vi "DualDigitalOscilloscope .vi"() -> ()   [LabVIEW 2014]
panel:
  out "error out":errorcluster
  in  "Digitalizing Parameters":T1={"Number of Samples"=500.0, "Sampling Frequency"=10000.0}
  out "Waveform Graph":dynamicdata(graph)=[{"t0"=timestamp(3496344962.5394974 s since 1904-01-01), "dt"=0.001, "Y"=[-8.590041558292159, -8.440717982918141, -8.128256863855041, -7.667459197369262, -7.046484650384645, -6.271253896732339, -5.352621206174619, -4.313939189246366, -3.190071979714034, -2.0010828273437613, -0.7699949874285559, 0.4729325219573479, 1.7063211765178325, 2.9114237139782557, 4.057652341722364, 5.131522209673436, 6.100800901298043, 6.935887140374739, 7.623953652074697, 8.147897360293387, 8.511665011024219, 8.741897737995128, 8.794851269409115, 8.618229869568173, 8.298864216063254, 7.82294041892513, 7.1825648838693406, 6.376750998367034, 5.423917425963085, 4.357612309823663, 3.198227557434465, 1.9710885457261196, 0.7107298974989072, -0.5670612807050067, -1.8261058143465623, -3.0483141536532927, -4.210334172626944, -5.280919877058353, -6.229811798823686, -7.034972944933502, -7.673050601942922, -8.14437327597263, -8.448611739372074, -8.592014997838334, -8.419996872667795, -8.09766857250493, -7.629963897237409, -7.000437829629278, -6.209748561703055, -5.274999584084324, -4.23006846068987, -3.0986365354251553, -1.9037271933812556, -0.6742839494635432, 0.5643677534595124, 1.7980852729994734, 3.0038455957522827, 4.145798472482477, 5.210459049692923, 6.168226131726614, 6.994431989489637, 7.665395522728377, 8.17848541510827, 8.536661705681254, 8.746831296754884, 8.782024016310597, 8.600797963268812, 8.275183139881786, 7.7874188129598965, 7.132242622368013, 6.320837389419934, 5.359123434243318, 4.280977800184256, 3.115672782320264, 1.8865603316684036, 0.6252149379831347, -0.6459982141425034, -1.9076740432758632, -3.1275801285284786, -4.282364325913564, -5.345714197156835, -6.2873702687108395, -7.0856244502299175, -7.7105459043309725, -8.171014692750107, -8.465385972144972, -8.581818893579578, -8.405853893022162, -8.078263098049806, -7.594442035759566, -6.9543910116649785, -6.153505719278386, -5.2194146130551, -4.166260930666212, -3.028908791319053, -1.8336706095754256, -0.6055430353271211, 0.6373843747078365, 1.8641948895180325, 3.06995519739159], "attributes"=variant("NI_ChannelName"=variant(string "Voltage a0"), "NI_UnitDescription"=variant(string "Volts"))}, {"t0"=timestamp(3496344962.5395093 s since 1904-01-01), "dt"=0.001, "Y"=[4.935824630663836, 4.926944236431562, 4.922010684084116, 4.922668491063619, 4.921681780594383, 4.922010684084116, 4.9328644992520925, 4.934509016702939, 4.93220669227184, 4.935495727173594, 4.935824630663836, 4.936153534154091, 4.936482437644358, 4.936482437644358, 4.936153534154091, 4.935495727173594, 4.935824630663836, 4.936482437644358, 4.923655201532963, 4.922339587573861, 4.922339587573861, 4.924641912002416, -3.107194306725333e-05, -3.107194306725333e-05, -3.107194306725333e-05, -3.107194306725333e-05, -0.00035997572978681974, -3.107194306725333e-05, -0.00035997572978681974, 0.00029783184360059403, -0.00035997572978681974, -0.0006888795165581156, -0.0006888795165581156, -0.0006888795165581156, -0.00035997572978681974, -0.0006888795165581156, -0.00035997572978681974, -3.107194306725333e-05, -0.00035997572978681974, -0.00035997572978681974, 0.00029783184360059403, -0.00035997572978681974, -0.00035997572978681974, 4.935824630663836, 4.935824630663836, 4.936811341134637, 4.936811341134637, 4.936482437644358, 4.935824630663836, 4.936482437644358, 4.935824630663836, 4.936153534154091, 4.922668491063619, 4.922339587573861, 4.924313008512587, 4.924313008512587, 4.925628622471978, 4.934509016702939, 4.93253559576196, 4.936482437644358, 4.936482437644358, 4.936482437644358, 4.936482437644358, 4.937140244624929, 4.936482437644358, -3.107194306725333e-05, -0.00035997572978681974, -0.00035997572978681974, -0.00035997572978681974, -0.00035997572978681974, -0.0006888795165581156, -0.00035997572978681974, -0.00035997572978681974, -3.107194306725333e-05, -0.00035997572978681974, -0.00035997572978681974, -0.00035997572978681974, -3.107194306725333e-05, -0.0006888795165581156, -0.00035997572978681974, -0.00035997572978681974, -0.00035997572978681974, -0.00035997572978681974, -0.00035997572978681974, -0.00035997572978681974, -0.0006888795165581156, 4.924970815492259, 4.925299718982112, 4.924313008512587, 4.924641912002416, 4.933851209722564, 4.933193402742238, 4.9328644992520925, 4.936153534154091, 4.936811341134637, 4.936482437644358, 4.937140244624929, 4.936811341134637, 4.936153534154091, 4.936482437644358], "attributes"=variant("NI_ChannelName"=variant(string "Voltage a1"), "NI_UnitDescription"=variant(string "Volts"))}]
  in  "Stop":bool
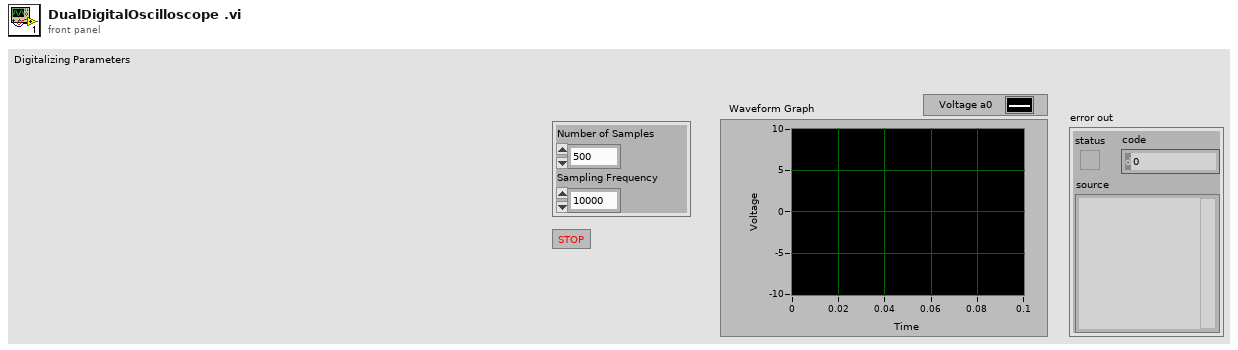
[diagram p1: front panel]
types:
  T1 = cluster{"Number of Samples":dbl, "Sampling Frequency":dbl}
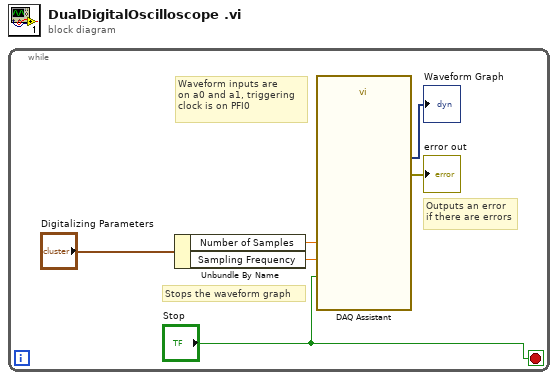
[diagram p0: block diagram]
diagram:
  n1 = while {
    stop <- "Stop" stop-if-true
    # "Waveform inputs are\non a0 and a1, triggering \nclock is on PFI0"
    # "Outputs an error \nif there are errors"
    # "Stops the waveform graph"
    n2 = Unbundle By Name("Digitalizing Parameters") -> ("Number of Samples"=w2:dbl, "Sampling Frequency"=w1:dbl)
    n3 = call "DAQ Assistant"("rate"=w1, "number of samples"=w2, "stop (T)"="Stop") -> ("data"=→"Waveform Graph":dynamicdata, "error out"=→"error out":errorcluster)  [unwired: 14 in, 1 out]
  }
